vi "Image.vi"(2 "XRef":refnum<vi>, 3 "State In":T1) -> (0 "Image":picture)   [LabVIEW 2012, in "Minimum Array Size.xnode"]
uses:
  Minimum Array Size.xnode
  State.ctl
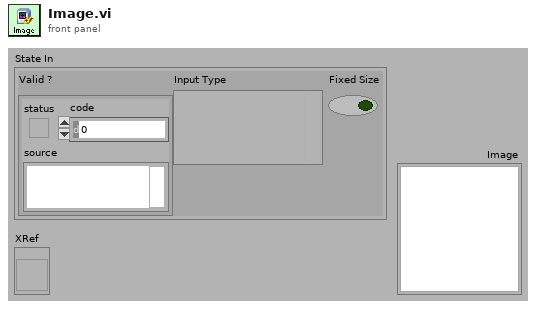
[diagram p1: front panel]
types:
  T1 = typedef "Minimum Array Size.xnode/State.ctl" = cluster{"Valid ?":errorcluster, "Input Type":variant, "Fixed Size":bool}
  T2 = typedef "imagedata.ctl" = cluster{"image type":i32, "image depth":i32, "image":u8[], "mask":u8[], "colors":u32[], "Rectangle":cluster{"left":i16, "top":i16, "right":i16, "bottom":i16}}
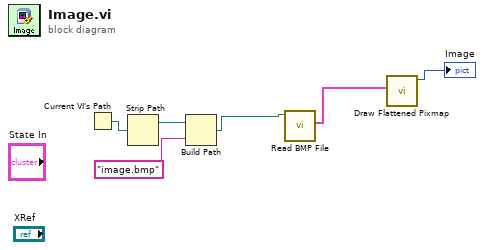
[diagram p0: block diagram]
diagram:
  n1 = Current VI's Path() -> (path=w5:path)
  n2 = Strip Path(path=w5) -> (stripped path=w4:path)  [unwired: 1 out]
  n3 = Build Path(base path=w4, name or relative path="image.bmp") -> (appended path=w2:path)
  n4 = call <vilib>:"Read BMP File.vi"("path to BMP file"=w2) -> ("image data"=w1:T2)  [unwired: 1 in, 9 out]
  n5 = call <vilib>:"Draw Flattened Pixmap.vi"("image data"=w1) -> ("new picture"=→"Image":picture)  [unwired: 1 in, 7 out]
